vi "Teleop Drivetrain Control.vi"(10 "Button Cluster":T1, 11 "Axes":T2) -> ()   [LabVIEW 2015]
uses:
  Common Code/Gamepads/Axes Cluster.ctl
  Common Code/Gamepads/Button Cluster.ctl
  Common Code/Drivetrain Modes.ctl
  Common Code/Shot Type.ctl
  Common Code/Change Detect.vi
  Common Code/Change Detect Boolean.vi
  Robot Global Data.vi
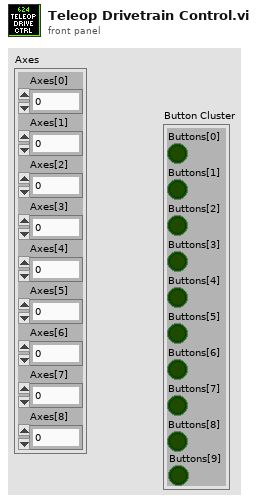
[diagram p1: front panel]
types:
  T1 = typedef "Button Cluster.ctl" = cluster{"Buttons[0]":bool, "Buttons[1]":bool, "Buttons[2]":bool, "Buttons[3]":bool, "Buttons[4]":bool, "Buttons[5]":bool, "Buttons[6]":bool, "Buttons[7]":bool, "Buttons[8]":bool, "Buttons[9]":bool}
  T2 = typedef "Axes Cluster.ctl" = cluster{"Axes[0]":dbl, "Axes[1]":dbl, "Axes[2]":dbl, "Axes[3]":dbl, "Axes[4]":dbl, "Axes[5]":dbl, "Axes[6]":dbl, "Axes[7]":dbl, "Axes[8]":dbl}
  T3 = typedef "Drivetrain Modes.ctl" = enum16{"Climb", "Manual", "Ball Vision Targeting", "Goal Vision Targeting", "PID Distance Drive", "Hybrid"}
  T4 = typedef "Shot Type.ctl" = enum16{"Batter Shot", "Curve Shot", "Vision Shot", "Deep Middle Shot"}
  T5 = typedef "Climb Command Cluster.ctl" = cluster{"Climb Mode":T6, "Hold?":bool, "Manual State":T7}
  T6 = typedef "Climb Mode.ctl" = enum16{"Auto", "Manual"}
  T7 = typedef "Climb Manual State.ctl" = cluster{"Release":bool, " PTO Engage":bool}
  T8 = typedef "Drivetrain Commands.ctl" = cluster{"Y Power":dbl, "Turn Power":dbl, "1st Gear?":bool, "Modes":T3, "Heading Target":dbl, "X Max Speed":dbl, "Y Max Speed":dbl, "X Min Speed":dbl, "Y Min Speed":dbl, "Y Target":dbl, "Max Accel":dbl, "Max Velocity":dbl}
  T9 = typedef "Shooter Command Cluster.ctl" = cluster{"Command":T10, "Mode":T11, "Shot Type":T4, "Override Trigger IR":bool}
  T10 = typedef "Shooter Commands.ctl" = enum16{"Idle", "Prime Shooter", "Shoot"}
  T11 = typedef "Shoot Modes Enum.ctl" = enum16{"Manual", "Safe", "Auto"}
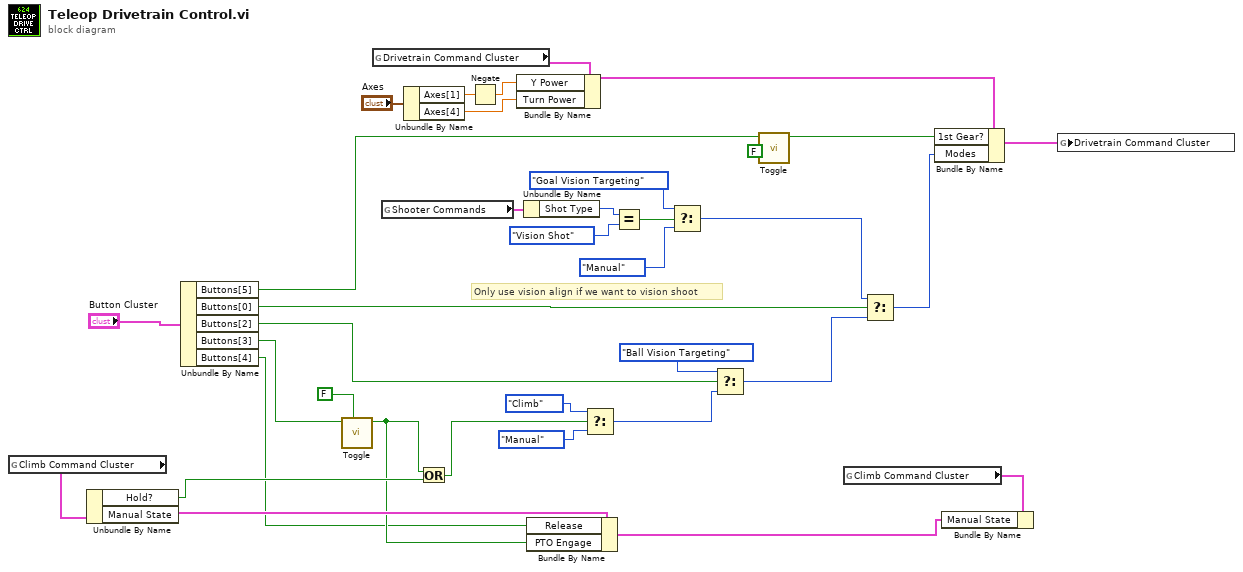
[diagram p0: block diagram]
diagram:
  # "Only use vision align if we want to vision shoot"
  n1 = global read "Robot Global Data.vi" "Climb Command Cluster"() -> (w7:T5)
  n2 = Unbundle By Name(w7) -> ("Hold?"=w6:bool, "Manual State"=w4:T7)
  n3 = Unbundle By Name("Button Cluster") -> ("Buttons[5]"=w31:bool, "Buttons[0]"=w22:bool, "Buttons[2]"=w24:bool, "Buttons[3]"=w13:bool, "Buttons[4]"=w2:bool)
  n4 = call "Toggle.vi"("Initial Value"=FALSE, "In"=w13) -> ("Toggled"=w3:bool)  [unwired: 9 in]
  n5 = global read "Robot Global Data.vi" "Drivetrain Command Cluster"() -> (w26:T8)
  n6 = global read "Robot Global Data.vi" "Shooter Commands"() -> (w20:T9)
  n7 = Unbundle By Name("Axes") -> ("Axes[1]"=w34:dbl, "Axes[4]"=w32:dbl)
  n8 = Or(x=w3, y=w6) -> (x .or. y?=w5:bool)
  n9 = Negate(x=w34) -> (-x=w33:dbl)
  n10 = Bundle By Name(cluster=w26, "Y Power"=w33, "Turn Power"=w32) -> (w29:T8)
  n11 = Unbundle By Name(w20) -> ("Shot Type"=w19:T4)
  n12 = Bundle By Name(cluster=w4, "Release"=w2, "PTO Engage"=w3) -> (w1:T7)
  n13 = Select(t=Drivetrain_Modes."Climb", s=w5, f=Drivetrain_Modes."Manual" ("Modes")) -> (s? t:f=w9:T3)
  n14 = Equal?(x=w19, y=Shot_Type."Vision Shot") -> (x = y?=w17:bool)
  n15 = Select(t=Drivetrain_Modes."Goal Vision Targeting" ("Modes"), s=w17, f=Drivetrain_Modes."Manual") -> (s? t:f=w14:T3)
  n16 = Select(t=Drivetrain_Modes."Ball Vision Targeting" ("Modes"), s=w24, f=w9) -> (s? t:f=w25:T3)
  n17 = call "Toggle.vi"("Initial Value"=FALSE, "In"=w31) -> ("Toggled"=w28:bool)  [unwired: 9 in]
  n18 = global read "Robot Global Data.vi" "Climb Command Cluster"() -> (w8:T5)
  n19 = Select(t=w14, s=w22, f=w25) -> (s? t:f=w21:T3)
  n20 = Bundle By Name(cluster=w29, "1st Gear?"=w28, "Modes"=w21) -> (w27:T8)
  n21 = Bundle By Name(cluster=w8, "Manual State"=w1) -> ()  [unwired: 1 out]
  n22 = global write "Robot Global Data.vi" "Drivetrain Command Cluster"(w27) -> ()
